vi "Robot Global Data.vi"() -> ()   [LabVIEW 2012]
doc: "This global VI can contain as many global variables as you need. Place a control on the panel, give it a good name. To read or write to it from a VI, drag the icon to the diagram of that VI. You can also drag from the project. Click on the node to change which global you access. You shouldn't have multiple locations writing to a global or it will cause a race-condition."
uses:
  <vilib>/Rock Robotics/WPI/Camera/WPI_CameraImageSize.ctl
  <vilib>/Rock Robotics/WPI/DriverStation/WPI_DriverStationRobotMode2.ctl
panel:
  in  "TeleopSeconds":dbl
  in  "Gyro 1 Angle":dbl min=0.0 max=360.0
  in  "Kinect Tracking":bool
  in  "BoxSpeed":T1
  in  "PickupState":T2(ring)
  in  "Actions":T3 {"Shooter" min=-1.0 max=1.0}
  in  "DIO":T4
  in  "Frisbee Count":i8 min=0 max=4 step=1
  in  "Robot Mode":T5
  out "Target Info":T6(array[cluster])
  in  "LED toggle rate (ms)":u32=20
  in  "image size":T7=enum."320x240"
  in  "Enable Vision":bool
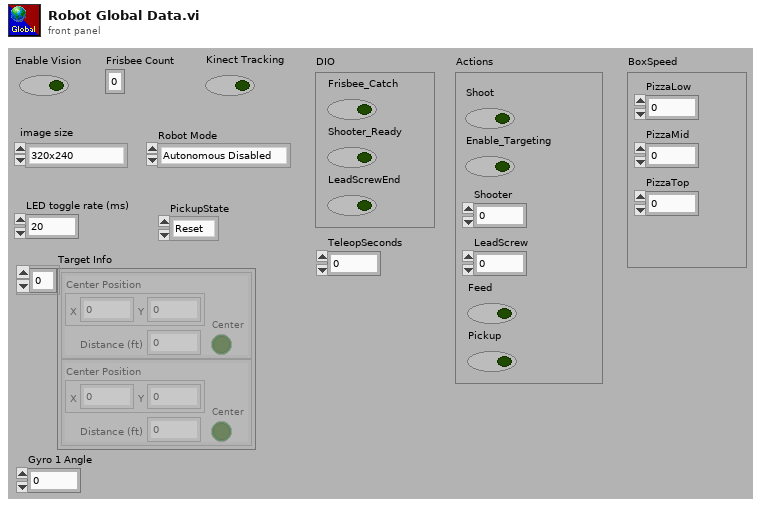
[diagram p1: front panel]
types:
  T1 = cluster{"PizzaLow":dbl, "PizzaMid":dbl, "PizzaTop":dbl}
  T2 = enum16{"Reset", "Ready", "Down", "Capture", "Lift", "Swing", "Release"}
  T3 = cluster{"Shoot":bool, "Enable_Targeting":bool, "Shooter":dbl, "LeadScrew":dbl, "Feed":bool, "Pickup":bool}
  T4 = cluster{"Frisbee_Catch":bool, "Shooter_Ready":bool, "LeadScrewEnd":bool}
  T5 = typedef "WPI_DriverStationRobotMode2.ctl" = enum16{"Autonomous Disabled", "Autonomous Enabled", "Teleop Disabled", "Teleop Enabled", "Timeout", "Finish", "Test Disabled", "Test Enabled"}
  T6 = cluster{"Center Position":cluster{"X":dbl, "Y":dbl}, "Distance (ft)":dbl, "Center":bool}[]
  T7 = typedef "WPI_CameraImageSize.ctl" = enum16{"640x480", "320x240", "160x120"}
diagram:
